vi "VI-Add File to Library.vi"(0 "LVClass.Create in":refnum<vi>, 5 "VI ref":refnum<vi>, 7 "Filename":string="Serialized.ctl", 11 "error in (no error)":errorcluster) -> (4 "reference out":refnum<vi>, 8 "file path":path, 15 "error out":errorcluster)   [LabVIEW 2020]
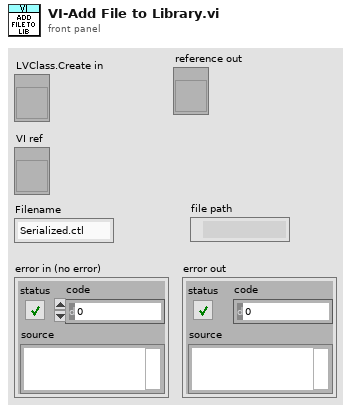
[diagram p1: front panel]
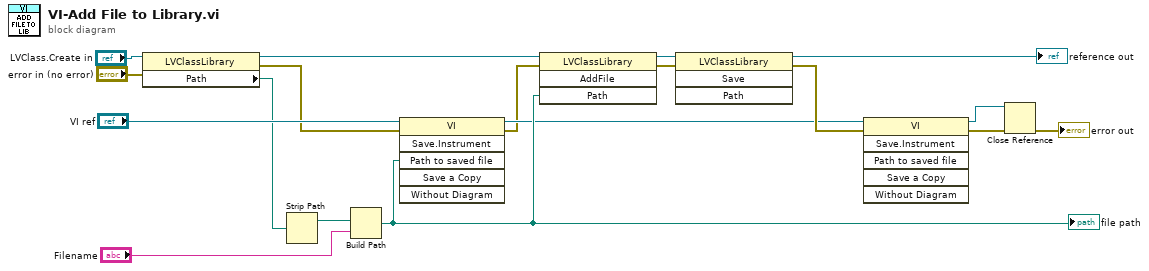
[diagram p0: block diagram]
diagram:
  n1 = property class="LVClassLibrary"(reference="LVClass.Create in", error in="error in (no error)") -> (reference out=w7:refnum<vi>, error out=w4:errorcluster, "Path"=w6:path)
  n2 = Strip Path(path=w6) -> (stripped path=w14:path)  [unwired: 1 out]
  n3 = Build Path(base path=w14, name or relative path="Filename") -> (appended path=w10:path)
  "file path" <- w10
  n4 = invoke class="VI" method="Save.Instrument"(reference="VI ref", error in=w4, "Path to saved file"=w10) -> (reference out=w8:refnum<vi>, error out=w3:errorcluster)  [unwired: 3 in, 4 out]
  n5 = invoke class="LVClassLibrary" method="AddFile"(reference=w7, error in=w3, "Path"=w10) -> (reference out=w18:refnum<vi>, error out=w16:errorcluster)  [unwired: 1 in, 2 out]
  n6 = invoke class="LVClassLibrary" method="Save"(reference=w18, error in=w16) -> (reference out=→"reference out":refnum<vi>, error out=w9:errorcluster)  [unwired: 2 in, 2 out]
  n7 = invoke class="VI" method="Save.Instrument"(reference=w8, error in=w9) -> (reference out=w11:refnum<vi>, error out=w13:errorcluster)  [unwired: 4 in, 4 out]
  n8 = Close Reference(reference=w11, error in (no error)=w13) -> (error out=→"error out":errorcluster)
